vi "Interface.vi"(0 "Data In":T4 {"time" format="%<%H:%M:%S%2u>T"}, 2 "Display State In":T2, 3 "Container State":T3) -> (6 "Data Out":T4 {"time" format="%<%H:%M:%S%2u>T"}, 7 "Display State Out":T2, 8 "Action":T1)   [LabVIEW 2015, in "Tau.xctl"]
uses:
  Tau.xctl
  Data.ctl
  <vilib>/_xctls/Container State.ctl
  State.ctl
  <vilib>/_xctls/Action.ctl
  <vilib>/_xctls/XControlSupport.lvlib
panel:
  out "Data":cluster{"Time Array":timestamp[], sgl[]}[](graph)
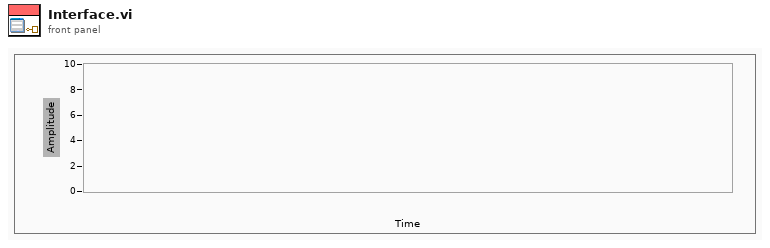
[diagram p1: front panel]
types:
  T1 = typedef "XControlSupport.lvlib/Action.ctl" = cluster{"Data Changed?":bool, "State Changed?":bool, "Action Name":string}
  T2 = typedef "Tau.xctl/State.ctl" = cluster{"Data Array":sgl[][], "Time Array":timestamp[], "History":u16, "Variable":bool[], "Plot Details":cluster{"Name":string, "Line Width":u8, "Line Style":u8, "Color":u32}[]}
  T3 = typedef "XControlSupport.lvlib/Container State.ctl" = cluster{"Indicator?":bool, "Run Mode?":bool, " Refnum":refnum<vi>}
  T4 = typedef "Tau.xctl/Data.ctl" = cluster{"time":timestamp, "data":sgl[]}
  T5 = cluster{"Name":string, "Line Width":u8, "Line Style":u8, "Color":u32}[]
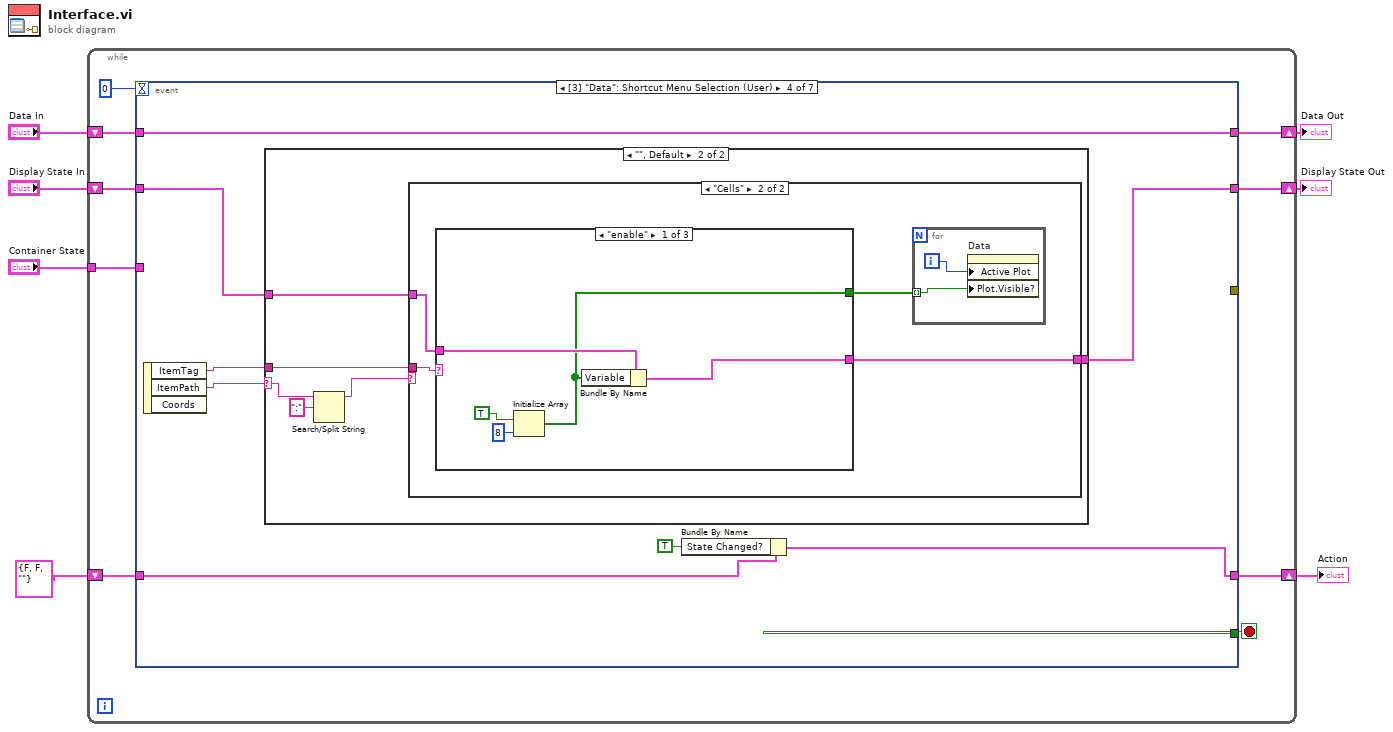
[diagram p0: block diagram]
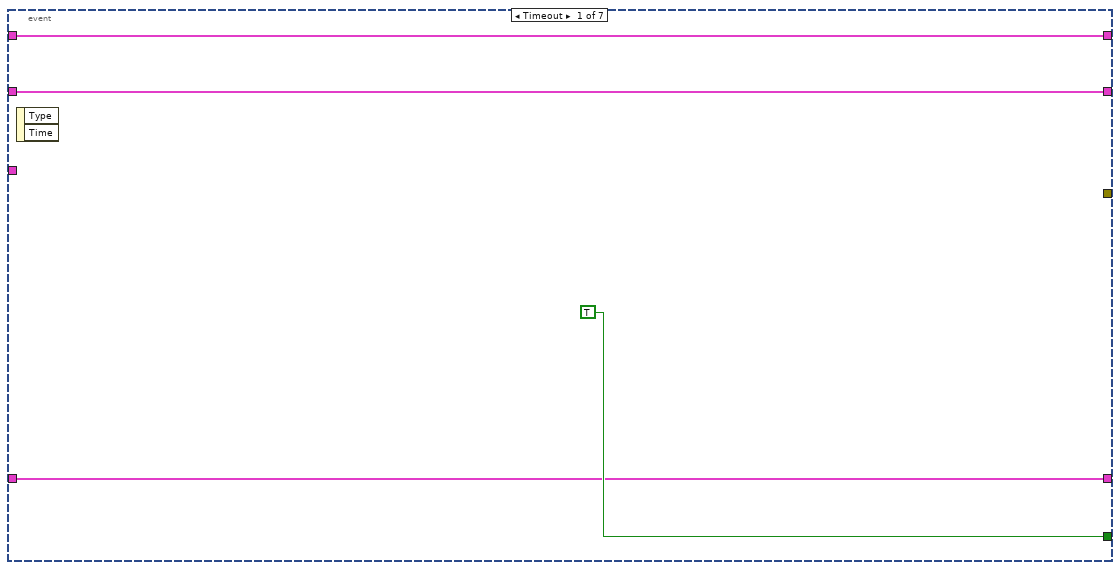
[diagram p2: hidden frame]
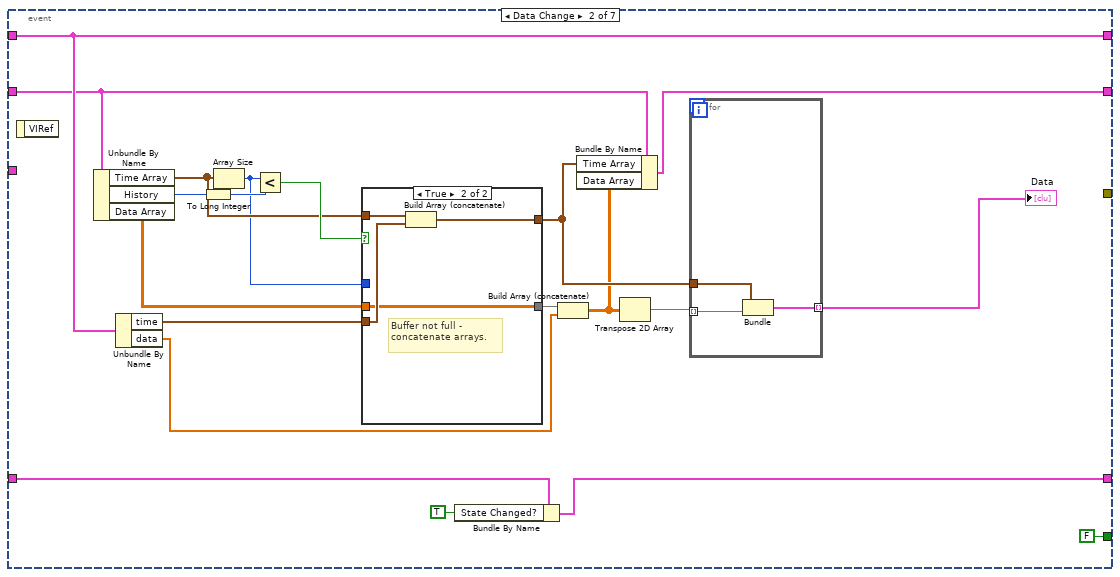
[diagram p3: hidden frame]
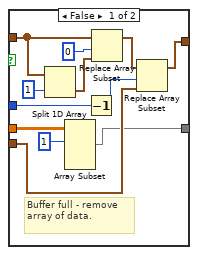
[diagram p4: hidden frame]
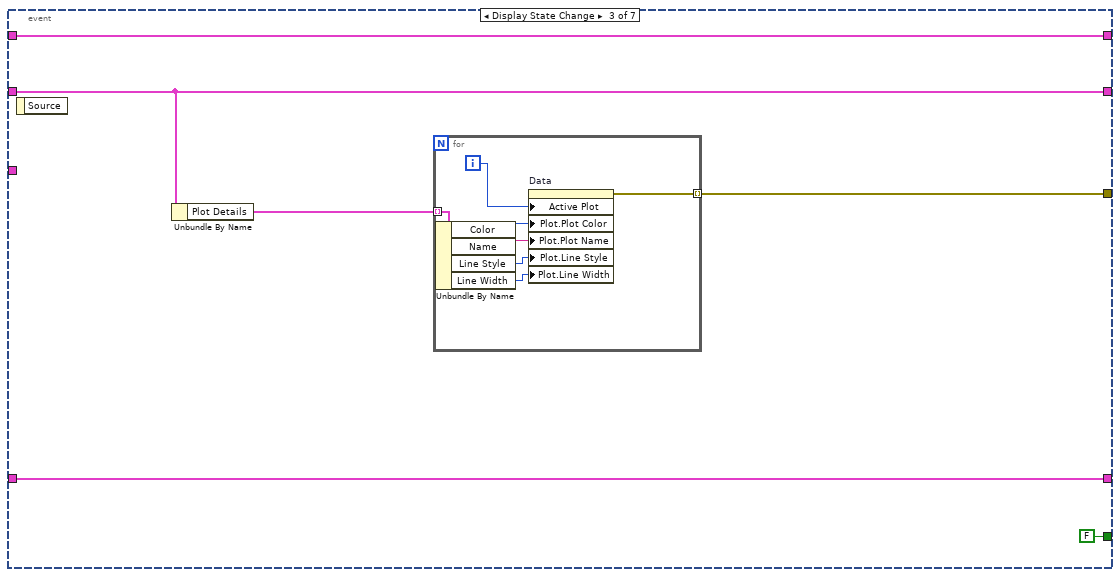
[diagram p5: hidden frame]
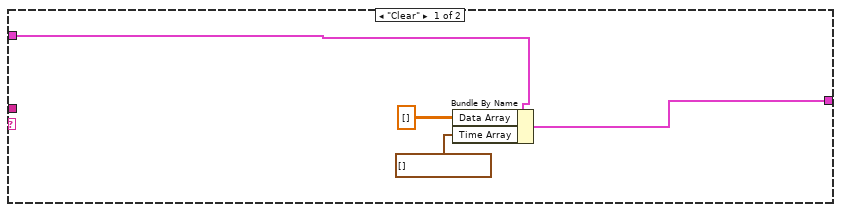
[diagram p6: hidden frame]
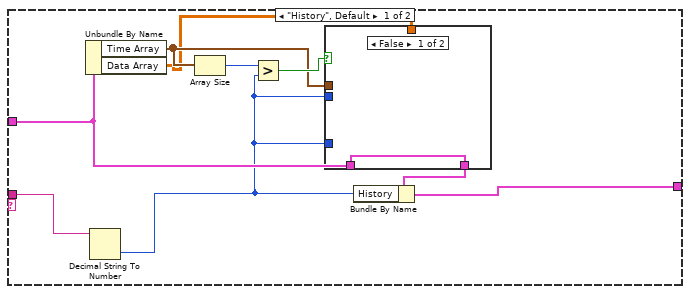
[diagram p7: hidden frame]
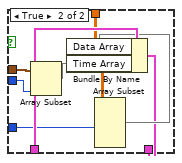
[diagram p8: hidden frame]
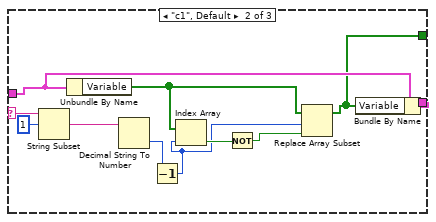
[diagram p9: hidden frame]
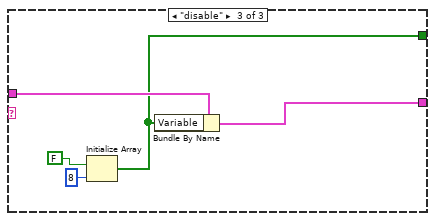
[diagram p10: hidden frame]
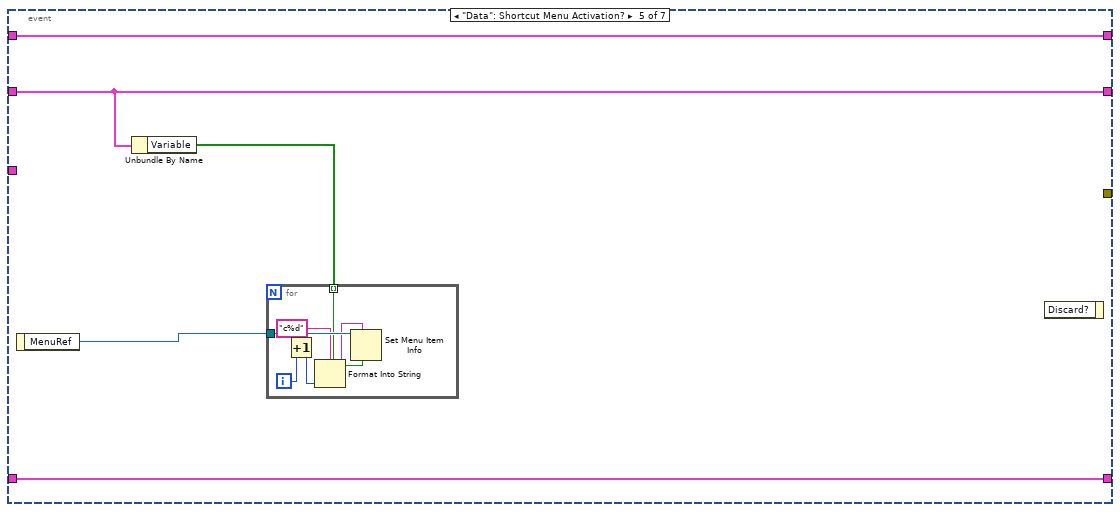
[diagram p11: hidden frame]
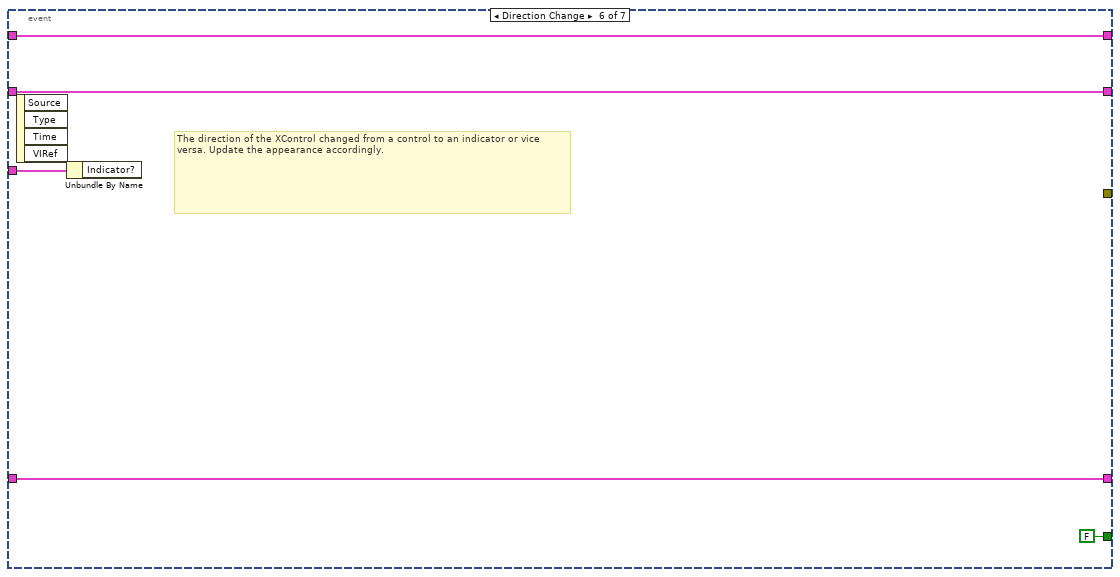
[diagram p12: hidden frame]
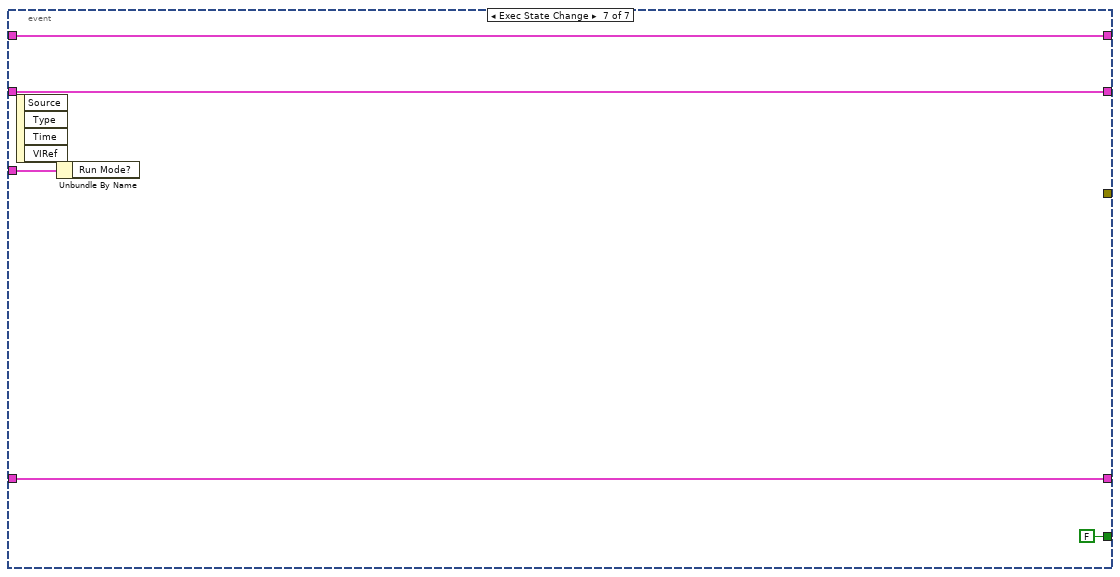
[diagram p13: hidden frame]
diagram:
  n1 = while {
    shift-right: [w15] -> w4
    shift-left: "Display State In" -> [w16]
    tunnel: "Container State" -> [w12]
    shift-right: [w10] -> w7
    shift-left: "Data In" -> [w11]
    shift-right: [w8] -> w2
    shift-left: T1 {"Data Changed?"=FALSE, "State Changed?"=FALSE, "Action Name"=""} ("Action") -> [w9]
    stop <- w14 stop-if-true
    n2 = event shown="[3] \"Data\": Shortcut Menu Selection (User)" {
      selector: _ -> [_ _ _ _ _ _ _]
      dyn-events: _ -> [_ _ _ _ _ _ _]
      timeout: 0 -> [_ _ _ _ _ _ _]
      tunnel: w16 -> [w18 w32 w62 w79 w137 w150 w152]
      tunnel: [w18 w31 w62 w78 w137 w150 w152] -> w15
      tunnel: [TRUE FALSE FALSE _ _ FALSE FALSE] -> w14
      tunnel: w12 -> [_ _ _ _ _ w151 w156]
      tunnel: w11 -> [w17 w40 w65 w80 w140 w149 w155]
      tunnel: [w17 w40 w65 w80 w140 w149 w155] -> w10
      tunnel: [w19 w27 w64 w75 w139 w148 w154] -> w8
      tunnel: w9 -> [w19 w29 w64 w77 w139 w148 w154]
      tunnel: [_ _ w60 _ _ _ _] -> _
      event Timeout {
        n3 = event-data() -> ()  [unwired: 1 in, 2 out]
      }
      event Data Change {
        n4 = event-data() -> ()  [unwired: 1 in, 1 out]
        n5 = Unbundle By Name(w32) -> ("Time Array"=w37:timestamp[], "History"=w39:u16, "Data Array"=w35:sgl[][])
        n6 = Unbundle By Name(w40) -> ("time"=w36:timestamp, "data"=w25:sgl[])
        n7 = To Long Integer(number=w39) -> (32bit integer=w34:i32)
        n8 = Array Size(array=w37) -> (size(s)=w33:i32)
        n9 = Less?(x=w33, y=w34) -> (x < y?=w38:bool)
        n10 = case shown="True" w38 {
          tunnel: w37 -> [w50 w59]
          tunnel: [w49 w57] -> w30
          tunnel: w36 -> [w48 w58]
          tunnel: w35 -> [w45 w56]
          tunnel: w33 -> [w47 _]
          tunnel: [w44 w56] -> w26
          frame False {
            # "Buffer full - remove array of data."
            n11 = Split 1D Array(array=w50, index=1) -> (second subarray=w51:timestamp[])  [unwired: 1 out]
            n12 = Array Subset(array=w45, index (row)=1 ("index")) -> (w44:sgl[][])  [unwired: 3 in]
            n13 = Decrement(x=w47) -> (x-1=w53:i32)
            n14 = Replace Array Subset(array=w50, new element=w51, index=0) -> (w54:timestamp[])
            n15 = Replace Array Subset(array=w54, new element=w48, index=w53) -> (w49:timestamp[])
          }
          frame True {
            # "Buffer not full - concatenate arrays."
            n16 = Build Array (concatenate)(w59, w58) -> (w57:timestamp[])
          }
        }
        n17 = Bundle By Name(cluster=w29, "State Changed?"=TRUE) -> (w27:T1)
        n18 = Build Array (concatenate)(w26, w25) -> (w23:sgl[][])
        n19 = Bundle By Name(cluster=w32, "Time Array"=w30, "Data Array"=w23) -> (w31:T2)
        n20 = Transpose 2D Array(2D array=w23) -> (transposed array=w24:sgl[][])
        n21 = for {
          tunnel: w30 -> [w43]
          tunnel: w24 -> [w42] mode=indexing
          tunnel: [w41] -> w21 mode=indexing
          n22 = Bundle("Time Array"=w43, w42) -> (w41:cluster{"Time Array":timestamp[], sgl[]})  [unwired: 1 in]
        }
        "Data" <- w21
      }
      event Display State Change {
        n23 = event-data() -> ()  [unwired: 1 in, 1 out]
        n24 = Unbundle By Name(w62) -> ("Plot Details"=w61:T5)
        n25 = for {
          tunnel: w61 -> [w71] mode=indexing
          tunnel: [w66] -> w60 mode=indexing
          i -> [w72]
          n26 = Unbundle By Name(w71) -> ("Color"=w70:u32, "Name"=w69:string, "Line Style"=w68:u8, "Line Width"=w67:u8)
          n27 = property on="Data" class="XYGraph (strict)"("Active Plot"=w72, "Plot.Plot Color"=w70, "Plot.Plot Name"=w69, "Plot.Line Style"=w68, "Plot.Line Width"=w67) -> (error out=w66:errorcluster)  [unwired: 2 in, 1 out]
        }
      }
      event "Data": Shortcut Menu Selection (User) {
        n28 = event-data() -> ("ItemTag"=w73:string, "ItemPath"=w74:string)  [unwired: 1 in, 1 out]
        n29 = case shown="\"\", Default" w74 {
          selector: w74 -> [_ w88]
          tunnel: w79 -> [w82 w90]
          tunnel: [w81 w89] -> w78
          tunnel: w73 -> [_ w85]
          frame "Clear" {
            n30 = Bundle By Name(cluster=w82, "Data Array"=sgl[][] [], "Time Array"=timestamp[] []) -> (w81:T2)
          }
          frame "", Default {
            n31 = Search/Split String(string=w88, search string/char (-)=":") -> (substring before match=w86:string)  [unwired: 1 in, 2 out]
            n32 = case shown="\"Cells\"" w86 {
              tunnel: w90 -> [w95 w112]
              tunnel: [w98 w111] -> w89
              tunnel: w85 -> [w99 w110]
              frame "History", Default {
                n33 = Unbundle By Name(w95) -> ("Time Array"=w94:timestamp[], "Data Array"=w93:sgl[][])
                n34 = Decimal String To Number(string=w99) -> (number=w92:i32)  [unwired: 2 in, 1 out]
                n35 = Array Size(array=w94) -> (size(s)=w97:i32)
                n36 = Greater?(x=w97, y=w92) -> (0:w96:bool)
                n37 = case shown="False" w96 {
                  tunnel: w95 -> [w100 w108]
                  tunnel: w94 -> [_ w107]
                  tunnel: w92 -> [_ w105]
                  tunnel: w93 -> [_ w104]
                  tunnel: w92 -> [_ w103]
                  tunnel: [w100 w101] -> w91
                  frame False {
                  }
                  frame True {
                    n38 = Array Subset(array=w107, length=w105) -> (w106:timestamp[])  [unwired: 1 in]
                    n39 = Array Subset(array=w104, length (row)=w103) -> (w102:sgl[][])  [unwired: 3 in]
                    n40 = Bundle By Name(cluster=w108, "Data Array"=w102, "Time Array"=w106) -> (w101:T2)
                  }
                }
                n41 = Bundle By Name(cluster=w91, "History"=w92) -> (w98:T2)
              }
              frame "Cells" {
                n42 = case shown="\"enable\"" w110 {
                  selector: w110 -> [_ w130 _]
                  tunnel: w112 -> [w119 w124 w133]
                  tunnel: [w116 w123 w132] -> w111
                  tunnel: [w115 w120 w131] -> w109
                  frame "enable" {
                    n43 = Initialize Array(TRUE, 8 ("dimension size")) -> (w115:bool[])
                    n44 = Bundle By Name(cluster=w119, "Variable"=w115) -> (w116:T2)
                  }
                  frame "c1", Default {
                    n45 = String Subset(string=w130, offset (0)=1) -> (substring=w128:string)  [unwired: 1 in]
                    n46 = Unbundle By Name(w124) -> ("Variable"=w126:bool[])
                    n47 = Decimal String To Number(string=w128) -> (number=w122:i32)  [unwired: 2 in, 1 out]
                    n48 = Decrement(x=w122) -> (x-1=w121:i32)
                    n49 = Index Array(array=w126, index=w121) -> (element=w127:bool)
                    n50 = Not(x=w127) -> (.not. x?=w125:bool)
                    n51 = Replace Array Subset(array=w126, new element=w125, index=w121) -> (w120:bool[])
                    n52 = Bundle By Name(cluster=w124, "Variable"=w120) -> (w123:T2)
                  }
                  frame "disable" {
                    n53 = Initialize Array(FALSE, 8 ("dimension size")) -> (w131:bool[])
                    n54 = Bundle By Name(cluster=w133, "Variable"=w131) -> (w132:T2)
                  }
                }
                n55 = for {
                  tunnel: w109 -> [w113] mode=indexing
                  i -> [w114]
                  n56 = property on="Data" class="XYGraph (strict)"("Active Plot"=w114, "Plot.Visible?"=w113) -> ()  [unwired: 2 in, 2 out]
                }
              }
            }
          }
        }
        n57 = Bundle By Name(cluster=w77, "State Changed?"=TRUE) -> (w75:T1)
      }
      event "Data": Shortcut Menu Activation? {
        n58 = event-data() -> ("MenuRef"=w138:refnum<k9>)  [unwired: 1 in]
        n59 = Unbundle By Name(w137) -> ("Variable"=w136:bool[])
        n60 = for {
          tunnel: w138 -> [w146]
          tunnel: w136 -> [w145] mode=indexing
          i -> [w144]
          n61 = Increment(x=w144) -> (x+1=w143:i32)
          n62 = Format Into String(format string="c%d", w143) -> (resulting string=w141:string)  [unwired: 2 in, 1 out]
          n63 = Set Menu Item Info(6:w145, 7:w141, 11:w146) -> ()  [unwired: 4 in, 2 out]
        }
        n64 = event-data() -> ()  [unwired: 2 in, 1 out]
      }
      event Direction Change {
        # "The direction of the XControl changed from a control to an indicator or vice versa. Update the appearance accordingly."
        n65 = event-data() -> ()  [unwired: 1 in, 4 out]
        n66 = Unbundle By Name(w151) -> ()  [unwired: 1 out]
      }
      event Exec State Change {
        n67 = event-data() -> ()  [unwired: 1 in, 4 out]
        n68 = Unbundle By Name(w156) -> ()  [unwired: 1 out]
      }
    }
  }
  "Display State Out" <- w4
  "Data Out" <- w7
  "Action" <- w2
